vi "Adjust_VI_Properties.vi"(6 "VI refnum in":refnum<vi>, 8 "error in (no error)":errorcluster, 9 "sourceInclusion":T3, 10 "properties in":T1[](array[typedef]), 11 "AB_PackedLibrary in":refnum<class "AB_PackedLibrary.lvclass">) -> (0 "error out":errorcluster, 1 "defaultSaveLevel":u32, 2 "properties out":T1[](array[typedef]), 3 "AB_PackedLibrary out":refnum<class "AB_PackedLibrary.lvclass">)   [LabVIEW 2020, in "AB_PackedLibrary.lvclass"]
uses:
  <vilib>/AppBuilder/AB_Classes/PackedLib/AB_PackedLibrary.lvclass
  <vilib>/AppBuilder/AB_Source_Properties.ctl
  <vilib>/AppBuilder/AB_Source_Property_Type.ctl
  e:/builds/penguin/labview/branches/2020/dev/dist/vi.lib/AppBuilder/AB_Classes/TargetFile/AB_Targetfile.lvclass
  <vilib>/AppBuilder/AB_Source_Inclusion.ctl
  <vilib>/AppBuilder/AB_Classes/TargetFile/AB_Targetfile.lvclass
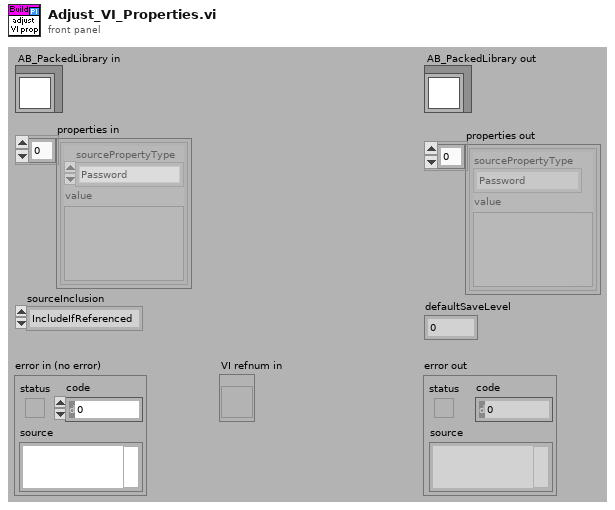
[diagram p1: front panel]
types:
  T1 = typedef "AB_Source_Properties.ctl" = cluster{"sourcePropertyType":T2, "value":variant}
  T2 = typedef "AB_Source_Property_Type.ctl" = enum16{"Remove block diagram", "Remove front panel", "Password", "Window has title bar", "Show menu bar", "Show vertical scroll bar", "Show horizontal scroll bar", "Show toolbar", "Show Abort button", "Show fp when called", "Window behavior", "Allow user to close window", "Window run-time position", "Run when opened", "Allow debugging", "Auto error handling", "Generate guard code", "Use stack variables", "Expression folding", "Integer only", "Inline subVI"}
  T3 = typedef "AB_Source_Inclusion.ctl" = enum16{"IncludeIfReferenced", "Include", "Exclude", "TopLevel"}
  T4 = enum32{"invalid scope", "public", "private", "protected", "community"}
  T5 = typedef "AB_Targetfile.ctl" = cluster{"targetfileName":string, "targetfileGUID":string, "enableDebugging":bool, "versionInfo":cluster{"productName":string, "legalCopyright":string, "companyName":string, "internalName":string, "fileDescription":string}, "eng_consolidatedTypeInfo":string, "fastFileFormat":bool, "eng_LEIFBuildData":u32, "versionIndependent":bool}
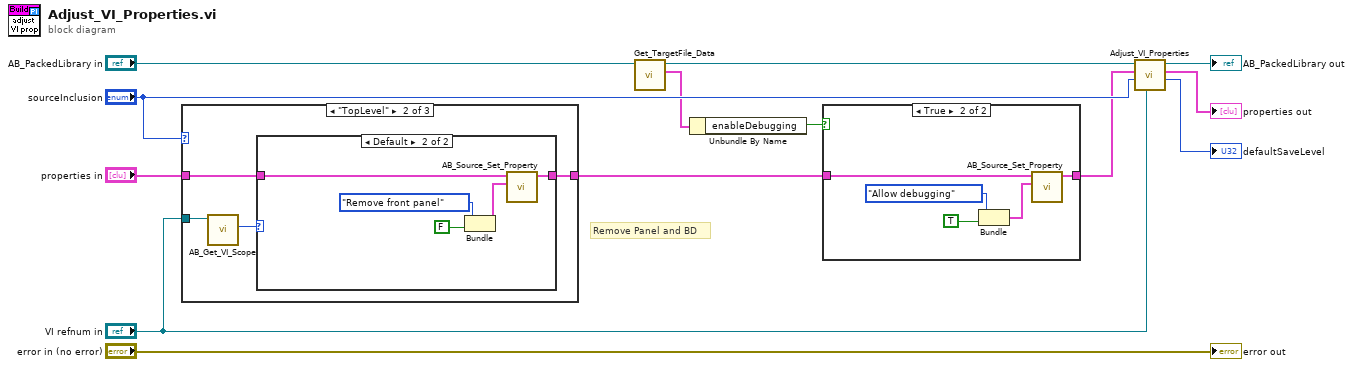
[diagram p0: block diagram]
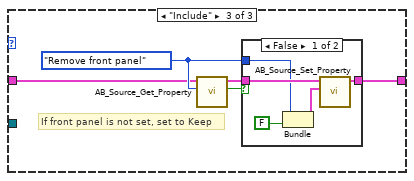
[diagram p5: hidden frame]
diagram:
  # "Remove Panel and BD"
  n1 = case shown="\"TopLevel\"" "sourceInclusion" {
    tunnel: "properties in" -> [w14 w18 w26]
    tunnel: [w14 w17 w25] -> w3
    tunnel: "VI refnum in" -> [_ w16 _]
    frame Default {
    }
    frame "TopLevel" {
      n2 = call <vilib>:"AB_Get_VI_Scope.vi"("vi reference"=w16) -> ("Source Scope"=w15:T4)  [unwired: 8 in, 2 out]
      n3 = case shown="Default" w15 {
        tunnel: w18 -> [w19 w22]
        tunnel: [w19 w20] -> w17
        frame "private" {
          # "The rule with packed libraries is that any VI that is part of the source library (which means its inclusion will be TopLevel) that is  scoped private will have its FP and BD removed by default.  So don't automatically keep it's front panel in this case."
        }
        frame Default {
          n4 = Bundle("sourcePropertyType"=AB_Source_Property_Type."Remove front panel", FALSE) -> (w21:cluster{"sourcePropertyType":T2, bool})  [unwired: 1 out]
          n5 = call <vilib>:"AB_Source_Set_Property.vi"("sourceProperty"=w21, "sourceProperties in"=w22) -> ("sourceProperties out"=w20:T1[])  [unwired: 1 in, 8 out]
        }
      }
    }
    frame "Include" {
      w27 = AB_Source_Property_Type."Remove front panel" ("sourcePropertyType")
      # "If front panel is not set, set to Keep"
      n6 = call <vilib>:"AB_Source_Get_Property.vi"("type"=w27, "sourceProperties in"=w26) -> ("found"=w29:bool, "sourceProperties out"=w28:T1[])  [unwired: 1 in, 7 out]
      n7 = case shown="False" w29 {
        tunnel: w28 -> [w34 w35]
        tunnel: [w33 w35] -> w25
        tunnel: w27 -> [w31 _]
        frame False {
          n8 = Bundle("sourcePropertyType"=w31, FALSE) -> (w30:cluster{"sourcePropertyType":T2, bool})  [unwired: 1 out]
          n9 = call <vilib>:"AB_Source_Set_Property.vi"("sourceProperty"=w30, "sourceProperties in"=w34) -> ("sourceProperties out"=w33:T1[])  [unwired: 1 in, 8 out]
        }
        frame True {
        }
      }
    }
  }
  n10 = call <vilib>:"Get_TargetFile_Data.vi"("AB_Targetfile in"="AB_PackedLibrary in") -> ("data"=w6:T5, "AB_Targetfile out"=w4:refnum<class "AB_PackedLibrary.lvclass">)  [unwired: 8 in, 1 out]
  n11 = Unbundle By Name(w6) -> ("enableDebugging"=w7:bool)
  n12 = case shown="True" w7 {
    tunnel: w3 -> [w36 w40]
    tunnel: [w36 w38] -> w2
    frame False {
    }
    frame True {
      n13 = Bundle("sourcePropertyType"=AB_Source_Property_Type."Allow debugging", TRUE) -> (w39:cluster{"sourcePropertyType":T2, bool})  [unwired: 1 out]
      n14 = call <vilib>:"AB_Source_Set_Property.vi"("sourceProperty"=w39, "sourceProperties in"=w40) -> ("sourceProperties out"=w38:T1[])  [unwired: 1 in, 8 out]
    }
  }
  n15 = call-parent "Adjust_VI_Properties.vi"("VI refnum in"="VI refnum in", "sourceInclusion"="sourceInclusion", "properties in"=w2, "AB_Targetfile in"=w4) -> ("defaultSaveLevel"=→"defaultSaveLevel":u32, "properties out"=→"properties out":T1[], "AB_Targetfile out"=→"AB_PackedLibrary out":refnum<class "AB_PackedLibrary.lvclass">)  [unwired: 1 in, 4 out]
  "error out" <- "error in (no error)"
